vi "MissingDependencies_Issue163.vi"   [LabVIEW 2013]
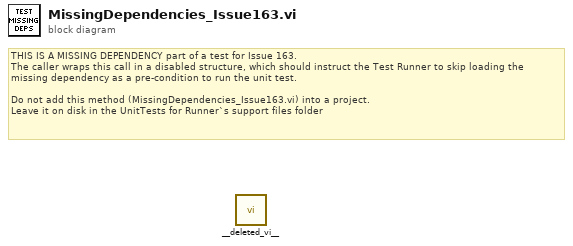
[diagram p0: block diagram]
diagram:
  # "THIS IS A MISSING DEPENDENCY part of a test for Issue 163.\nThe caller wraps this call in a disabled structure, which should instruct the Test Runner to skip loading the\nmissing dependency as a pre-condition to run the unit test.\n\nDo not add this method (MissingDependencies_Issue163.vi) into a project.\nLeave it on disk in the UnitTests for Runner`s support files folder"
  n1 = call "__deleted_vi__.vi"() -> ()  [unwired: 12 in]
